vi "Load LCOS Pattern.vi"(0 "Images Dest":T1, 3 "error in":errorcluster) -> (5 "Cancelled?":bool, 6 "Images Out":T1, 7 "Correct File Type":bool, 8 "Path":path, 9 "error out":errorcluster)   [LabVIEW 2011]
uses:
  LCOS Images.ctl
  <vilib>/vision/Image Controls.llb/IMAQ Image.ctl
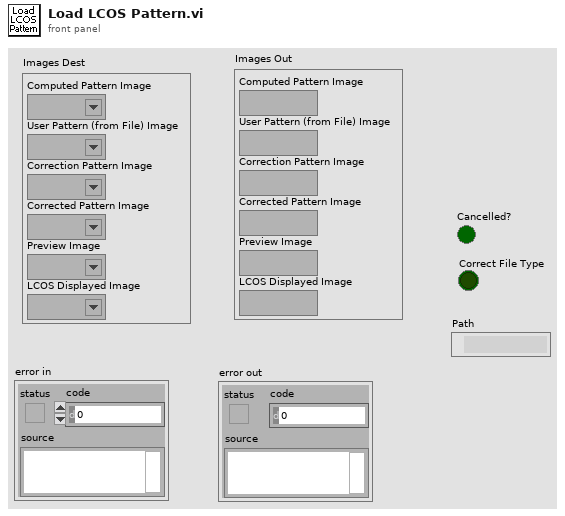
[diagram p1: front panel]
types:
  T1 = typedef "LCOS Images.ctl" = cluster{"Computed Pattern Image":T2, "User Pattern (from File) Image":T2, "Correction Pattern Image":T2, "Corrected Pattern Image":T2, "Preview Image":T2, "LCOS Displayed Image":T2}
  T2 = typedef "IMAQ Image.ctl" = refnum<image>
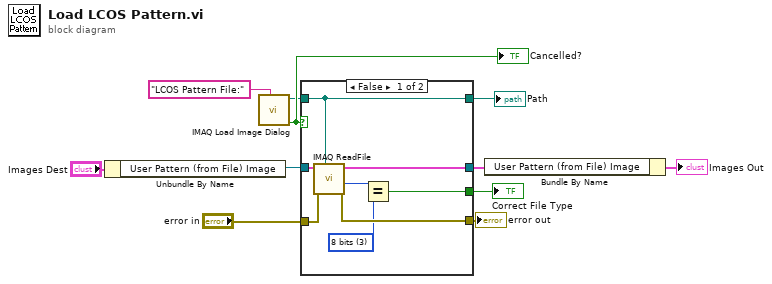
[diagram p0: block diagram]
diagram:
  n1 = Unbundle By Name("Images Dest") -> ("User Pattern (from File) Image"=w5:T2)
  n2 = call "IMAQ Load Image Dialog"("Prompt"="LCOS Pattern File:") -> ("Cancelled?"=w7:bool, "Path"=w6:path)  [unwired: 8 in, 1 out]
  "Cancelled?" <- w7
  n3 = case shown="False" w7 {
    tunnel: w5 -> [w19 w21]
    tunnel: [w18 w21] -> w3
    tunnel: "error in" -> [w17 w20]
    tunnel: [w16 w20] -> w10
    tunnel: [w14 _] -> w9
    tunnel: w6 -> [w12 _]
    tunnel: [w12 _] -> w1
    frame False {
      w13 = 3 items=["1 bit", "2 bits", "4 bits", "8 bits", "12 bits (unsigned)", "16 bits (unsigned)", "16 bits (signed)", "16 bits (RGB chunky)", "24 bits (RGB chunky)", "24 bits (RGB planar)", "32 bits (unsigned)", "32 bits (signed)", "32 bits (RGB chunky)", "32 bits (float)", "48 bits (Complex 2x24 int)", "64 bits (Complex 2x32 float)", "reserved", "24 bits (HSL)", "48 bits (RGB chunky)", "64 bits (RGB chunky)"] ("File Data Type")
      n4 = call "IMAQ ReadFile"("File Path"=w12, "error in (no error)"=w17, "Image"=w19) -> ("error out"=w16:errorcluster, "File Data Type out"=w15:i32, "Image Out"=w18:T2)  [unwired: 4 in, 2 out]
      n5 = Equal?(x=w15, y=w13) -> (x = y?=w14:bool)
    }
    frame True {
    }
  }
  "error out" <- w10
  "Correct File Type" <- w9
  "Path" <- w1
  n6 = Bundle By Name(cluster="Images Dest", "User Pattern (from File) Image"=w3) -> (→"Images Out":T1)
